vi "plot deaths and cases together.vi"(6 "country index":u16, 7 "SA data":T1, 8 "Countries (in)":string[](array[string]), 9 "US data":T1, 10 "deaths CSV":string[][](array[string]), 11 "cases CSV":string[][](array[string])) -> ()   [LabVIEW 2020]
panel:
  out "mortality rate":dbl
  out "Days ahead":i32
  in  "Country":u16(ring) items=["Afghanistan", "Albania", "Algeria", "Andorra", "Angola", "Antigua and Barbuda", "Argentina", "Armenia", "Australia, Australian Capital Territory", "Australia, New South Wales", "Australia, Northern Territory", "Australia, Queensland", "Australia, South Australia", "Australia, Tasmania", "Australia, Victoria", "Australia, Western Australia", "Austria", "Azerbaijan", "Bahamas", "Bahrain", "Bangladesh", "Barbados", "Belarus", "Belgium", "Benin", "Bhutan", "Bolivia", "Bosnia and Herzegovina", "Brazil", "Brunei", "Bulgaria", "Burkina Faso", "Cabo Verde", "Cambodia", "Cameroon", "Canada, Alberta", "Canada, British Columbia", "Canada, Grand Princess", "Canada, Manitoba", "Canada, New Brunswick", "Canada, Newfoundland and Labrador", "Canada, Nova Scotia", "Canada, Ontario", "Canada, Prince Edward Island", "Canada, Quebec", "Canada, Saskatchewan", "Central African Republic", "Chad", "Chile", "China, Anhui", "China, Beijing", "China, Chongqing", "China, Fujian", "China, Gansu", "China, Guangdong", "China, Guangxi", "China, Guizhou", "China, Hainan", "China, Hebei", "China, Heilongjiang", "China, Henan", "China, Hong Kong", "China, Hubei", "China, Hunan", "China, Inner Mongolia", "China, Jiangsu", "China, Jiangxi", "China, Jilin", "China, Liaoning", "China, Macau", "China, Ningxia", "China, Qinghai", "China, Shaanxi", "China, Shandong", "China, Shanghai", "China, Shanxi", "China, Sichuan", "China, Tianjin", "China, Tibet", "China, Xinjiang", "China, Yunnan", "China, Zhejiang", "Colombia", "Congo (Brazzaville)", "Congo (Kinshasa)", "Costa Rica", "Cote d'Ivoire", "Croatia", "Diamond Princess", "Cuba", "Cyprus", "Czechia", "Denmark, Faroe Islands", "Denmark, Greenland", "Denmark", "Djibouti", "Dominican Republic", "Ecuador", "Egypt", "El Salvador", "Equatorial Guinea", "Eritrea", "Estonia", "Eswatini", "Ethiopia", "Fiji", "Finland", "France, French Guiana", "France, French Polynesia", "France, Guadeloupe", "France, Mayotte", "France, New Caledonia", "France, Reunion", "France, Saint Barthelemy", "France, St Martin", "France, Martinique", "France", "Gabon", "Gambia", "Georgia", "Germany", "Ghana", "Greece", "Guatemala", "Guinea", "Guyana", "Haiti", "Holy See", "Honduras", "Hungary", "Iceland", "India", "Indonesia", "Iran", "Iraq", "Ireland", "Israel", "Italy", "Jamaica", "Japan", "Jordan", "Kazakhstan", "Kenya", "Korea South", "Kuwait", "Kyrgyzstan", "Latvia", "Lebanon", "Liberia", "Liechtenstein", "Lithuania", "Luxembourg", "Madagascar", "Malaysia", "Maldives", "Malta", "Mauritania", "Mauritius", "Mexico", "Moldova", "Monaco", "Mongolia", "Montenegro", "Morocco", "Namibia", "Nepal", "Netherlands, Aruba", "Netherlands, Curacao", "Netherlands, Sint Maarten", "Netherlands", "New Zealand", "Nicaragua", "Niger", "Nigeria", "North Macedonia", "Norway", "Oman", "Pakistan", "Panama", "Papua New Guinea", "Paraguay", "Peru", "Philippines", "Poland", "Portugal", "Qatar", "Romania", "Russia", "Rwanda", "Saint Lucia", "Saint Vincent and the Grenadines", "San Marino", "Saudi Arabia", "Senegal", "Serbia", "Seychelles", "Singapore", "Slovakia", "Slovenia", "Somalia", "South Africa", "Spain", "Sri Lanka", "Sudan", "Suriname", "Sweden", "Switzerland", "Taiwan*", "Tanzania", "Thailand", "Togo", "Trinidad and Tobago", "Tunisia", "Turkey", "Uganda", "Ukraine", "United Arab Emirates", "United Kingdom, Bermuda", "United Kingdom, Cayman Islands", "United Kingdom, Channel Islands", "United Kingdom, Gibraltar", "United Kingdom, Isle of Man", "United Kingdom, Montserrat", "United Kingdom", "Uruguay", "US", "Uzbekistan", "Venezuela", "Vietnam", "Zambia", "Zimbabwe", "Canada, Diamond Princess", "Dominica", "Grenada", "Mozambique", "Syria", "Timor-Leste", "Belize", "Laos", "Libya", "West Bank and Gaza", "Guinea-Bissau", "Mali", "Saint Kitts and Nevis", "Canada, Northwest Territories", "Canada, Yukon", "Kosovo", "Burma", "United Kingdom, Anguilla", "United Kingdom, British Virgin Islands", "United Kingdom, Turks and Caicos Islands", "MS Zaandam", "Botswana", "Burundi", "Sierra Leone", "Netherlands, \"Bonaire Sint Eustatius and Saba\"", "Malawi", "United Kingdom, Falkland Islands (Malvinas)", "France, Saint Pierre and Miquelon", "South Sudan", "Western Sahara", "Sao Tome and Principe", "Yemen", "Comoros", "Tajikistan", "Lesotho", "Australia", "Western Europe", "Latin America", "Africa", "China", "US and Canada", "US - Northeast", "US - Midwest", "US - South", "US - West", "Scandinavia (excl Sweden)", "Global", "South Asia", "South East Asia", "East Asia", "Eastern Europe and Russia", "Middle East", "Central Asia", "Canada", "American Samoa", "Guam", "Northern Mariana Islands", "Puerto Rico", "Virgin Islands", "Alabama", "Alaska", "Arizona", "Arkansas", "California", "Colorado", "Connecticut", "Delaware", "Florida", "Georgia", "Hawaii", "Idaho", "Illinois", "Indiana", "Iowa", "Kansas", "Kentucky", "Louisiana", "Maine", "Maryland", "Massachusetts", "Michigan", "Minnesota", "Mississippi", "Missouri", "Montana", "Nebraska", "Nevada", "New Hampshire", "New Jersey", "New Mexico", "New York", "North Carolina", "North Dakota", "Ohio", "Oklahoma", "Oregon", "Pennsylvania", "Rhode Island", "South Carolina", "South Dakota", "Tennessee", "Texas", "Utah", "Vermont", "Virginia", "Washington", "West Virginia", "Wisconsin", "Wyoming", "SA, EC", "SA, FS", "SA, GP", "SA, KZN", "SA, LP", "SA, MP", "SA, NC", "SA, NW", "SA, WC"]
  out "XY Graph":T2(graph)
  in  "Show mortality and days ahead":bool=TRUE
  in  "Data":enum16{"daily", "cumulative"}(ring)
  in  "Days":u16=7
  in  "Moving average":bool
  in  "Up/Down increment size":dbl=5.0 min=0.01 max=10.0
  in  "Down":bool
  in  "Up":bool
  in  "right":bool
  in  "left":bool
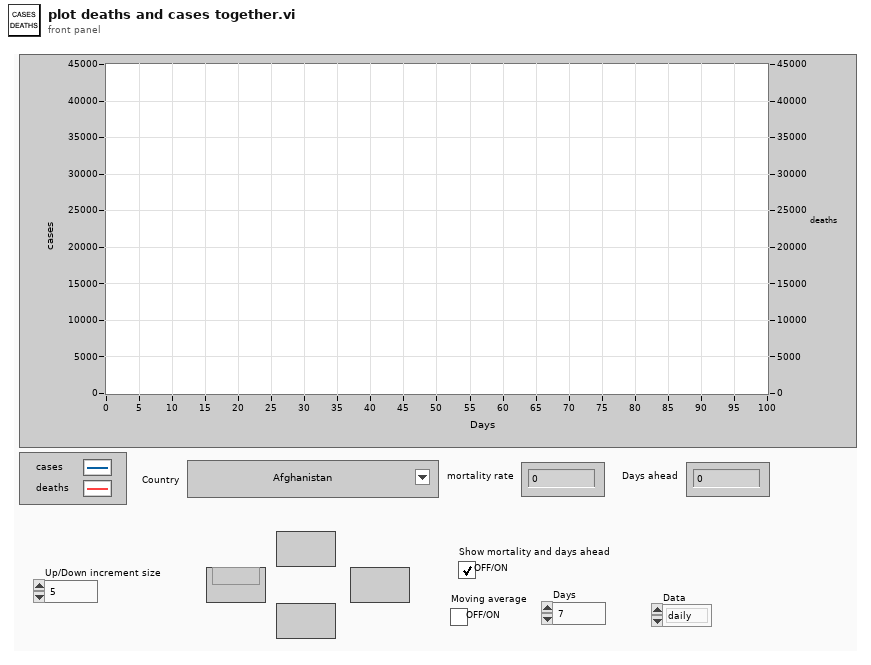
[diagram p1: front panel]
types:
  T1 = cluster{"cumulative deaths":i32[][], "deaths per day":i32[][], "case per day":i32[][], "cumulative cases":i32[][]}
  T2 = cluster{"cases days":i32[], "moving average array":dbl[]}[]
  T3 = cluster{"array index":i32[], "moving average array":dbl[]}
  T4 = cluster{"array index":i32[], "moving average array":dbl[]}[]
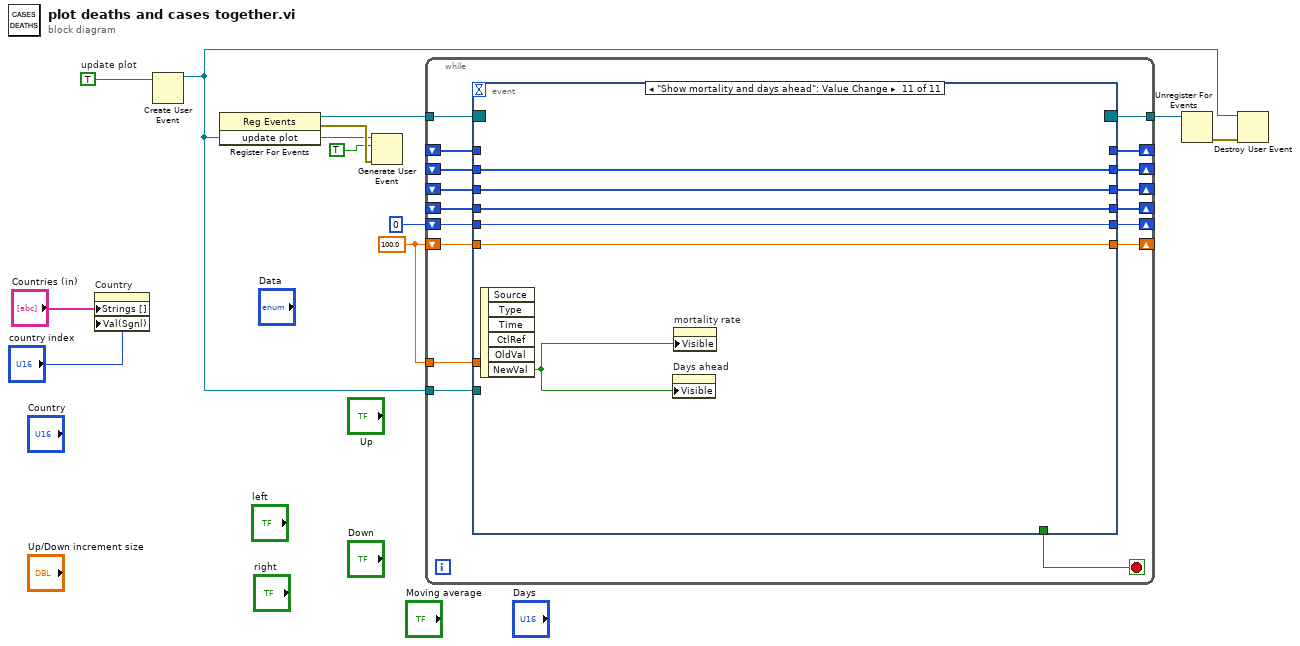
[diagram p0: block diagram]
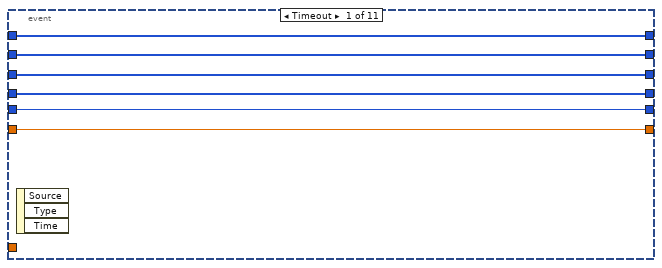
[diagram p2: hidden frame]
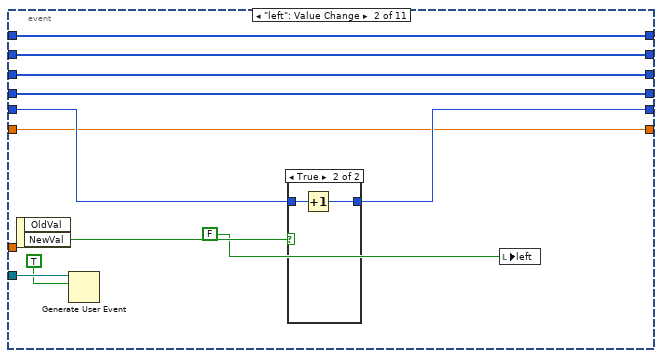
[diagram p3: hidden frame]
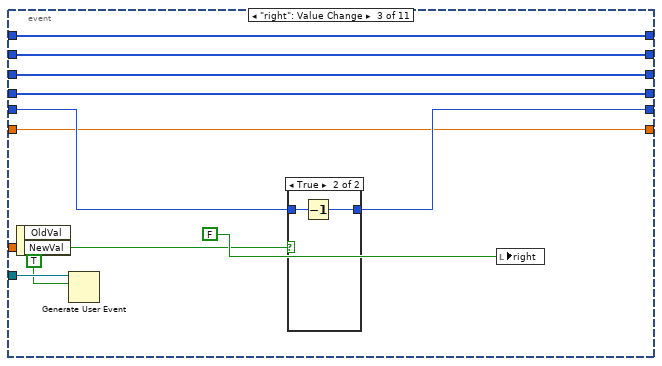
[diagram p5: hidden frame]
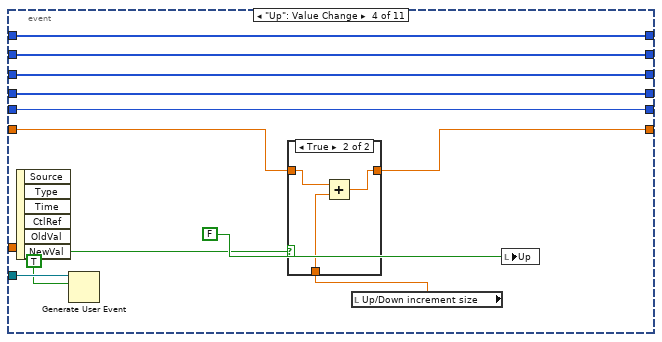
[diagram p7: hidden frame]
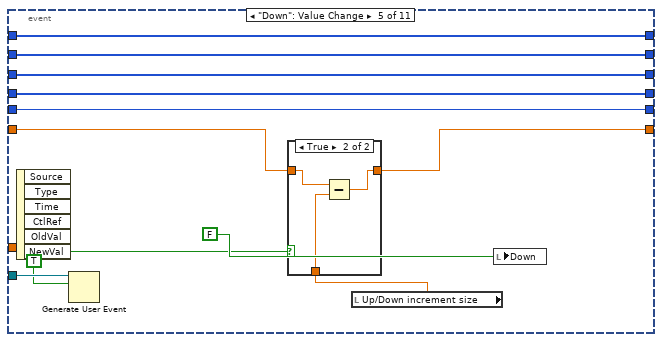
[diagram p9: hidden frame]
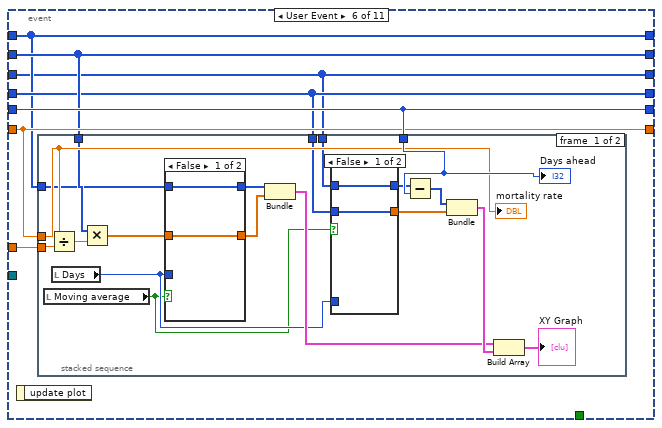
[diagram p11: hidden frame]
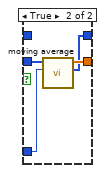
[diagram p12: hidden frame]
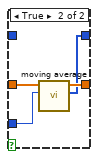
[diagram p13: hidden frame]
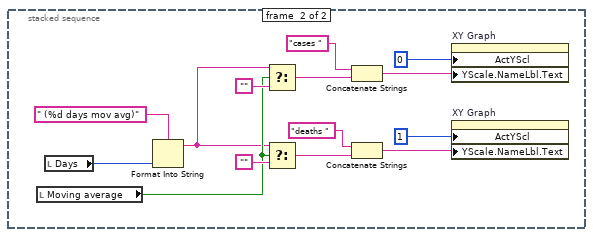
[diagram p14: hidden frame]
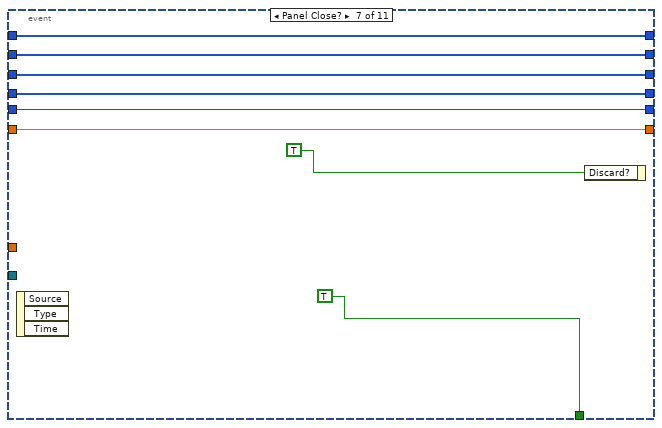
[diagram p15: hidden frame]
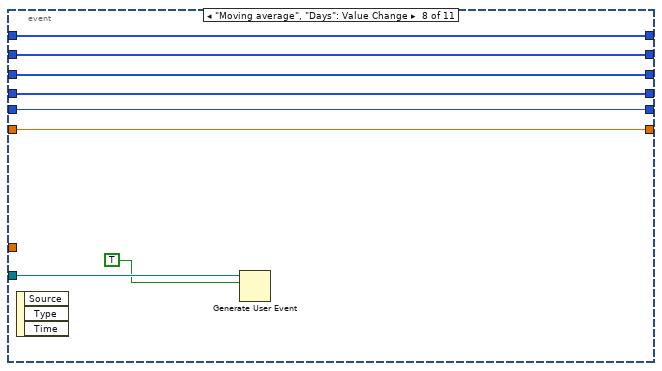
[diagram p16: hidden frame]
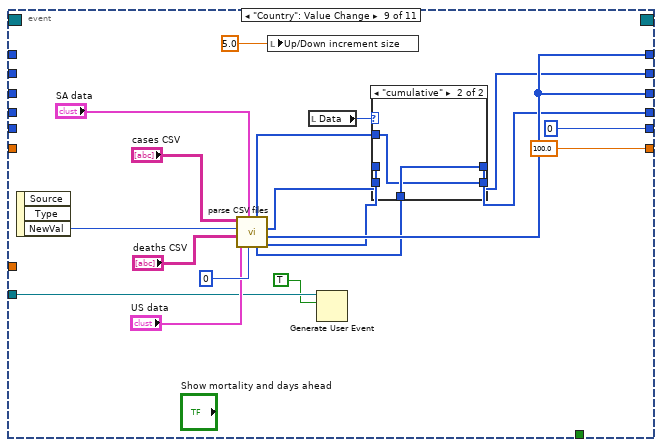
[diagram p17: hidden frame]
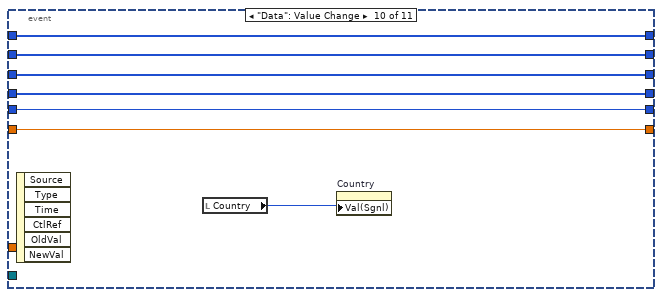
[diagram p19: hidden frame]
diagram:
  w7 = 100.0
  w9 = TRUE  # update plot
  n1 = property on="Country" class="Ring (strict)"("Strings []"="Countries (in)", "Val(Sgnl)"="country index") -> ()  [unwired: 2 in, 2 out]
  n2 = Create User Event(user event datatype=w9) -> (user event=w3:refnum<user-event>)  [unwired: 1 in, 1 out]
  n3 = register-events(w3) -> (reference out=w10:refnum<event-registration>, error out=w8:errorcluster)  [unwired: 2 in]
  n4 = Generate User Event(user event=w3, event data cluster=TRUE ("event data"), error in=w8) -> ()  [unwired: 1 in, 2 out]
  n5 = while {
    shift-right: [w24] -> _
    shift-left: _ -> [w28]
    shift-right: [w23] -> _
    shift-left: _ -> [w27]
    shift-right: [w21] -> _
    shift-left: _ -> [w26]
    shift-right: [w22] -> _
    shift-left: _ -> [w25]
    shift-right: [w19] -> _
    shift-left: 0 -> [w20]
    tunnel: w10 -> [w18]
    tunnel: w3 -> [w17]
    shift-right: [w15] -> _
    shift-left: w7 -> [w16]
    tunnel: w7 -> [w14]
    tunnel: [w12] -> w5
    stop <- w13 stop-if-true
    n6 = event shown="[10] \"Show mortality and days ahead\": Value Change" {
      selector: w18 -> [_ _ _ _ _ _ _ _ _ _ _]
      dyn-events: [_ _ _ _ _ _ _ _ _ _ _] -> w12
      timeout: _ -> [_ _ _ _ _ _ _ _ _ _ _]
      tunnel: w28 -> [w34 w45 w59 w74 w90 w96 w147 w155 _ w187 _]
      tunnel: w27 -> [w33 w44 w58 w73 w89 w98 w154 w162 _ w192 w198]
      tunnel: w26 -> [w31 w43 w57 w72 w88 w97 w152 w160 _ w190 w196]
      tunnel: w25 -> [w32 w42 w56 w71 w87 w95 w153 w161 _ w191 w197]
      tunnel: [w34 w45 w59 w74 w90 w96 w147 w155 w177 w187 _] -> w24
      tunnel: [w33 w44 w58 w73 w89 w98 w154 w162 w165 w192 w198] -> w23
      tunnel: [w32 w42 w56 w71 w87 w95 w153 w161 w177 w191 w197] -> w22
      tunnel: [w31 w43 w57 w72 w88 w97 w152 w160 w167 w190 w196] -> w21
      tunnel: w20 -> [w30 w41 w55 w66 w82 w100 w151 w159 _ w189 w195]
      tunnel: [w30 w40 w54 w66 w82 w100 w151 w159 0 w189 w195] -> w19
      tunnel: w17 -> [_ w38 w53 w70 w86 _ _ w157 w173 _ _]
      tunnel: w16 -> [w29 w35 w49 w65 w81 w99 w150 w158 _ w188 w194]
      tunnel: [w29 w35 w49 w63 w79 w99 w150 w158 100.0 w188 w194] -> w15
      tunnel: w14 -> [_ _ _ _ _ w101 _ _ _ _ _]
      tunnel: [_ _ _ _ _ _ TRUE _ _ _ _] -> w13
      event Timeout {
        n7 = event-data() -> ()  [unwired: 1 in, 3 out]
      }
      event "left": Value Change {
        n8 = event-data() -> ("NewVal"=w39:bool)  [unwired: 1 in, 1 out]
        n9 = Generate User Event(user event=w38, event data cluster=TRUE ("event data")) -> ()  [unwired: 2 in, 2 out]
        n10 = case shown="True" w39 {
          tunnel: w41 -> [w46 w48]
          tunnel: [w46 w47] -> w40
          frame False {
          }
          frame True {
            n11 = Increment(x=w48) -> (x+1=w47:i32)
          }
        }
        n12 = local write "left"(FALSE ("Previous Button")) -> ()
      }
      event "right": Value Change {
        n13 = event-data() -> ("NewVal"=w50:bool)  [unwired: 1 in, 1 out]
        n14 = Generate User Event(user event=w53, event data cluster=TRUE ("event data")) -> ()  [unwired: 2 in, 2 out]
        n15 = case shown="True" w50 {
          tunnel: w55 -> [w60 w62]
          tunnel: [w60 w61] -> w54
          frame False {
          }
          frame True {
            n16 = Decrement(x=w62) -> (x-1=w61:i32)
          }
        }
        n17 = local write "right"(FALSE ("Previous Button")) -> ()
      }
      event "Up": Value Change {
        n18 = event-data() -> ("NewVal"=w67:bool)  [unwired: 1 in, 5 out]
        n19 = Generate User Event(user event=w70, event data cluster=TRUE ("event data")) -> ()  [unwired: 2 in, 2 out]
        n20 = local read "Up/Down increment size"() -> (w64:dbl)
        n21 = case shown="True" w67 {
          tunnel: w65 -> [w75 w78]
          tunnel: [w75 w77] -> w63
          tunnel: w64 -> [_ w76]
          frame False {
          }
          frame True {
            n22 = Add(x=w78, y=w76) -> (x+y=w77:dbl)
          }
        }
        n23 = local write "Up"(FALSE ("Previous Button")) -> ()
      }
      event "Down": Value Change {
        n24 = event-data() -> ("NewVal"=w83:bool)  [unwired: 1 in, 5 out]
        n25 = Generate User Event(user event=w86, event data cluster=TRUE ("event data")) -> ()  [unwired: 2 in, 2 out]
        n26 = local read "Up/Down increment size"() -> (w80:dbl)
        n27 = case shown="True" w83 {
          tunnel: w81 -> [w91 w94]
          tunnel: [w91 w93] -> w79
          tunnel: w80 -> [_ w92]
          frame False {
          }
          frame True {
            n28 = Subtract(x=w94, y=w92) -> (x-y=w93:dbl)
          }
        }
        n29 = local write "Down"(FALSE ("Previous Button")) -> ()
      }
      event User Event {
        n30 = event-data() -> ()  [unwired: 1 in, 1 out]
        n31 = stacked-sequence {
          tunnel: w101 -> [w116 _]
          tunnel: w100 -> [w114 _]
          tunnel: w99 -> [w113 _]
          tunnel: w98 -> [w112 _]
          tunnel: w97 -> [w109 _]
          tunnel: w96 -> [w106 _]
          tunnel: w95 -> [w104 _]
          frame #0 {
            n32 = local read "Moving average"() -> (w102:bool)
            n33 = Divide(x=w113, y=w116) -> (x/y=w115:dbl)
            n34 = local read "Days"() -> (w107:u16)
            n35 = Multiply(x=w112, y=w115) -> (x*y=w111:dbl[])
            n36 = case shown="False" w102 {
              tunnel: w111 -> [w127 w132]
              tunnel: [w127 w131] -> w110
              tunnel: w107 -> [_ w130]
              tunnel: w106 -> [w128 _]
              tunnel: [w128 w129] -> w105
              frame False {
              }
              frame True {
                n37 = call "moving average.vi"("average over x points"=w130, "Array"=w132) -> ("array index"=w129:i32[], "moving average array"=w131:dbl[])  [unwired: 8 in]
              }
            }
            n38 = Bundle("array index"=w105, "moving average array"=w110) -> (w119:T3)  [unwired: 1 in]
            n39 = case shown="False" w102 {
              tunnel: w109 -> [w121 w126]
              tunnel: [w121 w125] -> w108
              tunnel: w107 -> [_ w124]
              tunnel: w104 -> [w122 _]
              tunnel: [w122 w123] -> w103
              frame False {
              }
              frame True {
                n40 = call "moving average.vi"("average over x points"=w124, "Array"=w126) -> ("array index"=w123:i32[], "moving average array"=w125:dbl[])  [unwired: 8 in]
              }
            }
            n41 = Subtract(x=w103, y=w114) -> (x-y=w118:i32[])
            n42 = Bundle(w118, "moving average array"=w108) -> (w120:cluster{i32[], "moving average array":dbl[]})  [unwired: 1 in]
            n43 = Build Array(w119, w120) -> (→"XY Graph":T4)
            "Days ahead" <- w114
            "mortality rate" <- w113
          }
          frame #1 {
            n44 = local read "Moving average"() -> (w135:bool)
            n45 = local read "Days"() -> (w134:u16)
            n46 = Format Into String(format string=" (%d days mov avg)", w134) -> (resulting string=w133:string)  [unwired: 2 in, 1 out]
            n47 = Select(t=w133, s=w135, f="") -> (s? t:f=w144:string)
            n48 = Select(t=w133, s=w135, f="") -> (s? t:f=w145:string)
            n49 = Concatenate Strings("cases " ("Y Scale.Name Label.Text"), w144) -> (w143:string)
            n50 = Concatenate Strings("deaths " ("Y Scale.Name Label.Text"), w145) -> (w146:string)
            n51 = property on="XY Graph" class="XYGraph (strict)"("ActYScl"=0 ("Active Y Scale"), "YScale.NameLbl.Text"=w143) -> ()  [unwired: 2 in, 2 out]
            n52 = property on="XY Graph" class="XYGraph (strict)"("ActYScl"=1 ("Active Y Scale"), "YScale.NameLbl.Text"=w146) -> ()  [unwired: 2 in, 2 out]
          }
        }
      }
      event Panel Close? {
        n53 = event-data() -> ()  [unwired: 1 in, 3 out]
        n54 = event-data("Discard?"=TRUE) -> ()  [unwired: 1 in, 1 out]
      }
      event "Moving average", "Days": Value Change {
        n55 = event-data() -> ()  [unwired: 1 in, 3 out]
        n56 = Generate User Event(user event=w157, event data cluster=TRUE ("event data")) -> ()  [unwired: 2 in, 2 out]
      }
      event "Country": Value Change {
        n57 = event-data() -> ("NewVal"=w180:u16)  [unwired: 1 in, 2 out]
        n58 = call "parse CSV files.vi"("threshold cases"=u32 0, "SA data"="SA data", "US data"="US data", "deaths CSV"="deaths CSV", "country index"=w180, "cases CSV"="cases CSV") -> ("new deaths per day"=w168:i32[], "days"=w177:i32[], "new cases per day"=w166:i32[], "cumulative cases"=w163:i32[], "cumulative deaths"=w164:i32[])  [unwired: 1 out]
        n59 = local write "Up/Down increment size"(5.0 ("Up/Down increment size")) -> ()
        n60 = local read "Data"() -> (w169:enum16{"daily", "cumulative"})
        n61 = Generate User Event(user event=w173, event data cluster=TRUE ("event data")) -> ()  [unwired: 2 in, 2 out]
        n62 = case shown="\"cumulative\"" w169 {
          tunnel: w168 -> [w183 _]
          tunnel: [w183 w184] -> w167
          tunnel: w166 -> [w182 _]
          tunnel: [w182 w185] -> w165
          tunnel: w164 -> [_ w184]
          tunnel: w163 -> [_ w185]
          frame "daily", Default {
          }
          frame "cumulative" {
          }
        }
      }
      event "Data": Value Change {
        n63 = event-data() -> ()  [unwired: 1 in, 6 out]
        n64 = local read "Country"() -> (w186:u16)
        n65 = property on="Country" class="Ring (strict)"("Val(Sgnl)"=w186) -> ()  [unwired: 2 in, 2 out]
      }
      event "Show mortality and days ahead": Value Change {
        n66 = event-data() -> ("NewVal"=w193:bool)  [unwired: 1 in, 5 out]
        n67 = property on="Days ahead" class="DigNum (strict)"("Visible"=w193) -> ()  [unwired: 2 in, 2 out]
        n68 = property on="mortality rate" class="DigNum (strict)"("Visible"=w193) -> ()  [unwired: 2 in, 2 out]
      }
    }
  }
  n69 = Unregister For Events(event registration refnum=w5) -> (error out=w4:errorcluster)  [unwired: 1 in]
  n70 = Destroy User Event(user event=w3, error in=w4) -> ()  [unwired: 1 out]
